vi "Cmd_Q(MS).vi"(0 "VISA resource name IN":refnum<visa-resource-name>) -> (1 "Position 1":string, 3 "Position 2":string, 4 "VISA resource name OUT":refnum<visa-resource-name>, 8 "OK Done":bool, 11 "Q String":string, 12 "Position 4":string, 14 "Positon 3":string, 15 "error out":errorcluster)   [LabVIEW 2011]
panel:
  out "Status":string
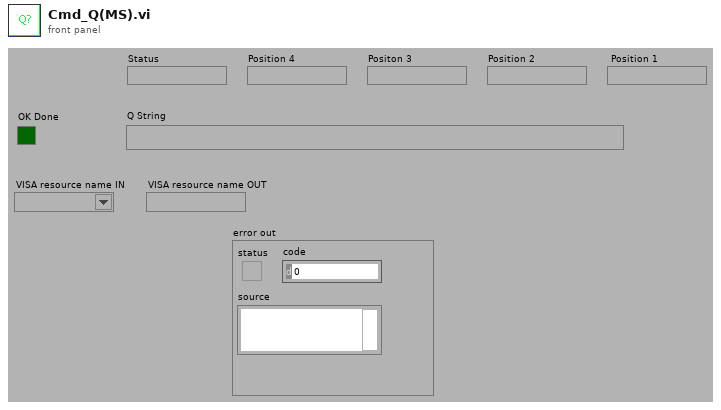
[diagram p1: front panel]
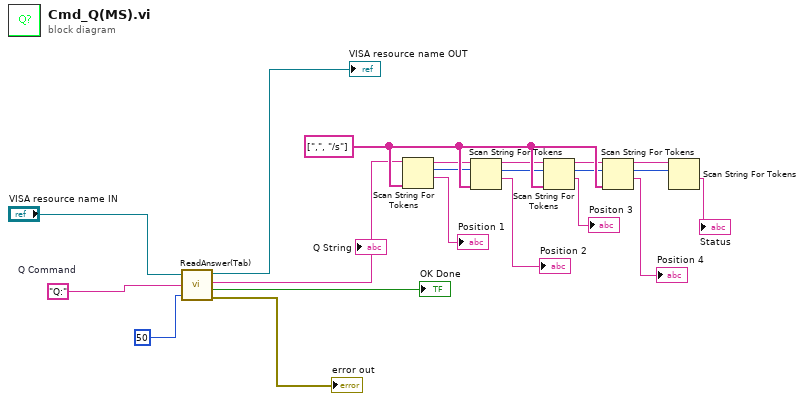
[diagram p0: block diagram]
diagram:
  w19 = "Q:"  # Q Command
  w21 = string[] [",", "/s"] ("delimiters (\\s,\\t,\\r,\\n)")
  n1 = call "ReadAnswer(Tab).vi"("Bytes to Read"=u32 50, "Command (\\r is appended)"=w19, "VRN IN"="VISA resource name IN") -> ("error out"=→"error out":errorcluster, "OKdone"=→"OK Done":bool, "String Received"=w5:string, "VRN OUT"=→"VISA resource name OUT":refnum<visa-resource-name>)
  "Q String" <- w5
  n2 = Scan String For Tokens(6:w21, 9:w5) -> (1:→"Position 1":string, 2:w7:i32, 3:w8:string)  [unwired: 4 in, 1 out]
  n3 = Scan String For Tokens(6:w21, 8:w7, 9:w8) -> (1:→"Position 2":string, 2:w11:i32, 3:w10:string)  [unwired: 3 in, 1 out]
  n4 = Scan String For Tokens(6:w21, 8:w11, 9:w10) -> (1:→"Positon 3":string, 2:w13:i32, 3:w12:string)  [unwired: 3 in, 1 out]
  n5 = Scan String For Tokens(6:w21, 8:w13, 9:w12) -> (1:→"Position 4":string, 2:w15:i32, 3:w14:string)  [unwired: 3 in, 1 out]
  n6 = Scan String For Tokens(8:w15, 9:w14) -> (1:→"Status":string)  [unwired: 4 in, 3 out]
